vi "practice.vi"() -> ()   [LabVIEW 2023]
uses:
  Control 1.ctl
  <vilib>/DAQmx/read.llb/DAQmx Read (Analog Wfm 1Chan NSamp).vi
  <vilib>/DAQmx/write.llb/DAQmx Write (Analog DBL 1Chan 1Samp).vi
  <extravilib>/ChannelInstances/Stream-c(bool,i32,str)/Read With Abort.vi
  <extravilib>/ChannelInstances/Stream-bool/Read With Abort.vi
  <extravilib>/ChannelInstances/Stream-bool/Write With Abort.vi
  <extravilib>/ChannelInstances/Stream-c(bool,i32,str)/Write With Abort.vi
  <extravilib>/ChannelInstances/Stream-c(bool,i32,str)/EndpointRead.vi
  <extravilib>/ChannelInstances/Stream-bool/EndpointRead.vi
  <extravilib>/ChannelInstances/Stream-bool/Endpoint.vi
  <extravilib>/ChannelInstances/Stream-c(bool,i32,str)/Endpoint.vi
  <vilib>/DAQmx/create/channels.llb/DAQmx Create Channel (AO-Voltage-Basic).vi
  <vilib>/DAQmx/configure/timing.llb/DAQmx Timing (Sample Clock).vi
  <vilib>/DAQmx/create/channels.llb/DAQmx Create Channel (AI-Voltage-Basic).vi
  <extravilib>/ChannelInstances/Stream-c(bool,i32,str)/Instantiate.vi
  <extravilib>/ChannelInstances/Stream-bool/Instantiate.vi
  <extravilib>/ChannelInstances/Stream-c(bool,i32,str)/)Channel.vi
  <resource>/ChannelSupport/_ChannelSupport/WaitIfNeeded.vi
  <extravilib>/ChannelInstances/Stream-bool/)Channel.vi
  <vilib>/DAQmx/miscellaneous.llb/DAQmx Fill In Error Info.vi
  <extravilib>/ChannelInstances/Stream-c(bool,i32,str).lvlib
  <extravilib>/ChannelInstances/Stream-bool.lvlib
panel:
  out "error out":errorcluster
  in  "Collection Parameters 2":T1={"physical channels"="", "samples per channel"=1000, "rate"=1000.0} {"rate" format="%0.2f"}
  out "error out 3":errorcluster
  out "Waveform Chart 2":waveform(dbl)(graph)
  in  "Collection Parameters":T1={"physical channels"="", "samples per channel"=1000, "rate"=1000.0} {"rate" format="%0.2f"}
  out "error out 2":errorcluster
  out "Waveform Chart":u32(graph)
  in  "stop":bool
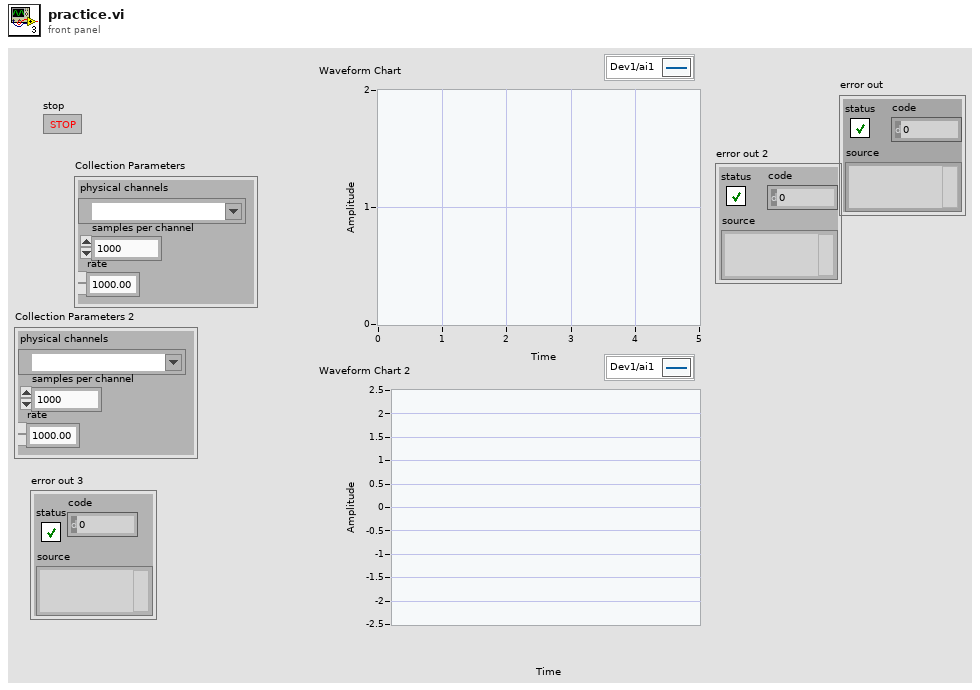
[diagram p1: front panel]
types:
  T1 = typedef "Control 1.ctl" = cluster{"physical channels":tag, "samples per channel":i32, "rate":dbl}
  T2 = typedef "Stream-bool.lvlib/)Channel.ctl" = refnum<queue>
  T3 = typedef "Stream-c(bool,i32,str).lvlib/)Channel.ctl" = refnum<queue>
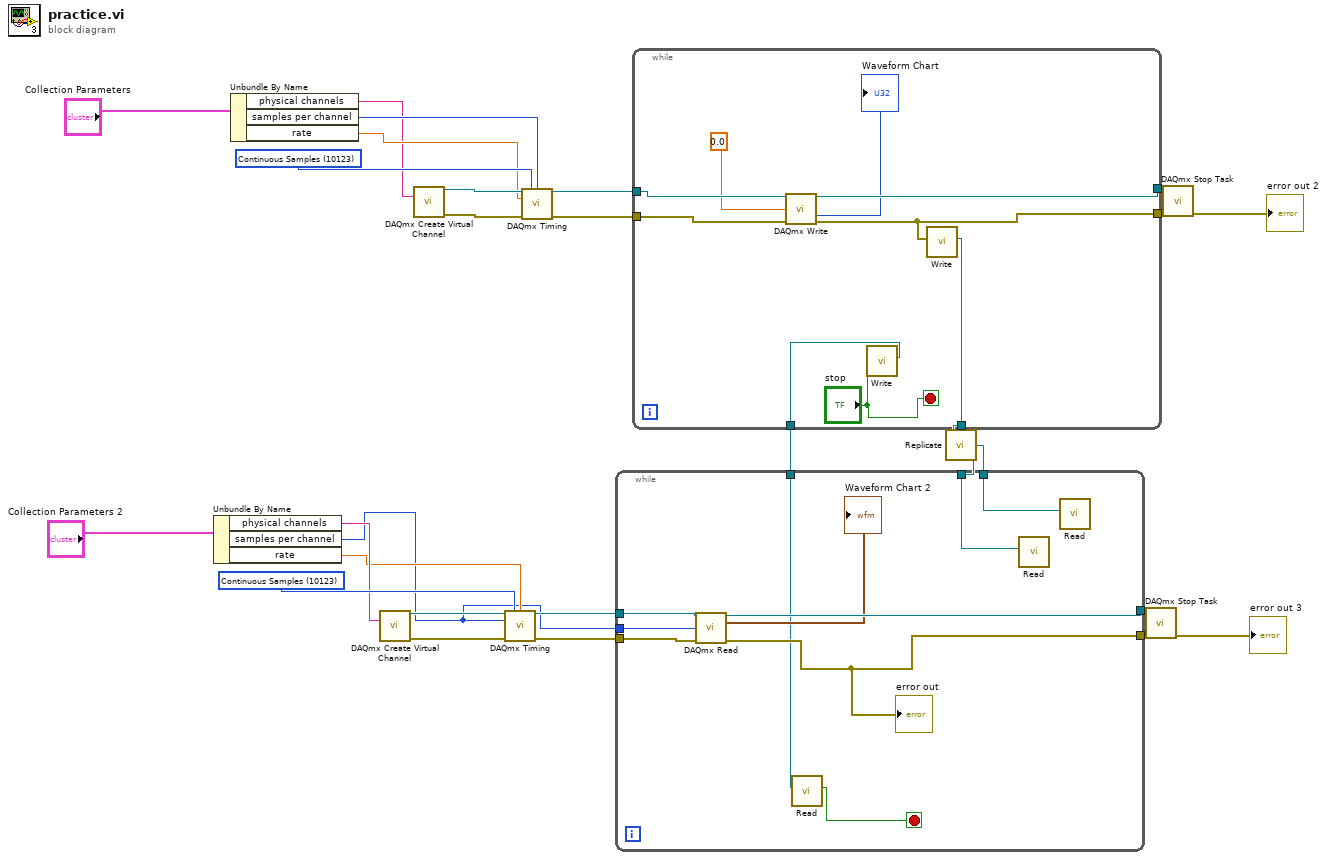
[diagram p0: block diagram]
diagram:
  w13 = 10123 items=["Finite Samples"=10178, "Continuous Samples"=10123, "Hardware Timed Single Point"=12522] ("sample mode")
  w22 = 10123 items=["Finite Samples"=10178, "Continuous Samples"=10123, "Hardware Timed Single Point"=12522] ("sample mode")
  n1 = Unbundle By Name("Collection Parameters 2") -> ("physical channels"=w10:tag, "samples per channel"=w8:i32, "rate"=w9:dbl)
  n2 = Unbundle By Name("Collection Parameters") -> ("physical channels"=w3:tag, "samples per channel"=w4:i32, "rate"=w5:dbl)
  n3 = call-poly <vilib>:"DAQmx Create Virtual Channel.vi"("physical channels"=w10) -> ("task out"=w19:refnum<k21>, "error out"=w18:errorcluster)  [unwired: 13 in]
  n4 = call-poly <vilib>:"DAQmx Create Virtual Channel.vi"("physical channels"=w3) -> ("task out"=w28:refnum<k21>, "error out"=w27:errorcluster)  [unwired: 13 in]
  n5 = call-poly <vilib>:"DAQmx Timing.vi"("task/channels in"=w19, "sample mode"=w13, "samples per channel"=w9, "rate"=w8, "error in"=w18) -> ("task out"=w17:refnum<k21>, "error out"=w16:errorcluster)  [unwired: 9 in]
  n6 = call-poly <vilib>:"DAQmx Timing.vi"("task/channels in"=w28, "sample mode"=w22, "samples per channel"=w4, "rate"=w5, "error in"=w27) -> ("task out"=w26:refnum<k21>, "error out"=w25:errorcluster)  [unwired: 9 in]
  n7 = while {
    tunnel: w26 -> [w32]
    tunnel: w25 -> [w36]
    tunnel: [w35] -> w24
    tunnel: [w34] -> w23
    tunnel: [w31] -> w7
    tunnel: [w30] -> w6
    stop <- "stop" stop-if-true
    n8 = call-poly <vilib>:"DAQmx Write.vi"("task/channels in"=w32, "data"=0.0, "error in"=w36) -> ("task out"=w35:refnum<k21>, "number of samples written per channel"=→"Waveform Chart":u32, "error out"=w34:errorcluster)  [unwired: 10 in]
    n9 = call <extravilib>:"Write.vi"("element"="stop") -> ("channel"=w30:T2)  [unwired: 8 in, 2 out]
    n10 = call <extravilib>:"Write.vi"("element"=w34) -> ("channel"=w31:T3)  [unwired: 8 in, 2 out]
  }
  n11 = call <extravilib>:"Replicate.vi"("stream"=w7) -> ("stream copy 1"=w1:T3, "stream copy 2"=w2:T3)  [unwired: 7 in]
  n12 = while {
    tunnel: w17 -> [w45]
    tunnel: w16 -> [w47]
    tunnel: [w44] -> w15
    tunnel: [w42] -> w14
    tunnel: w8 -> [w46]
    tunnel: w2 -> [w41]
    tunnel: w6 -> [w40]
    tunnel: w1 -> [w38]
    stop <- w39 stop-if-true
    n13 = call-poly <vilib>:"DAQmx Read.vi"("task/channels in"=w45, "number of samples per channel"=w46, "error in"=w47) -> ("task out"=w44:refnum<k21>, "data"=→"Waveform Chart 2":waveform(dbl), "error out"=w42:errorcluster)  [unwired: 10 in]
    "error out" <- w42
    n14 = call <extravilib>:"Read.vi"("channel"=w40) -> ("element"=w39:bool)  [unwired: 6 in, 4 out]
    n15 = call <extravilib>:"Read.vi"("channel"=w41) -> ()  [unwired: 6 in, 5 out]
    n16 = call <extravilib>:"Read.vi"("channel"=w38) -> ()  [unwired: 6 in, 5 out]
  }
  n17 = call <vilib>:"DAQmx Stop Task.vi"("task/channels in"=w15, "error in"=w14) -> ("error out"=→"error out 3":errorcluster)  [unwired: 12 in, 1 out]
  n18 = call <vilib>:"DAQmx Stop Task.vi"("task/channels in"=w24, "error in"=w23) -> ("error out"=→"error out 2":errorcluster)  [unwired: 12 in, 1 out]
